vi "TSM Set AI Microphone DAQmx Tasks.vi"(0 "TSM context":T1, 5 "Sampling Rate (Hz)":dbl format="%#_6pHz", 7 "Samples per channel":i32=1000, 9 "max dB SPL":dbl=132.0 format="%.2p", 11 "error in (no error)":errorcluster) -> (15 "error out":errorcluster)   [LabVIEW 2020]
doc: "Use this VI to initialize AI tasks for Microphones on connected NI-DAQmx instruments in the pin map associated with the test program."
uses:
  <vilib>/NI_TestStand_SemiconductorModule/NI_TestStand_Semiconductor_Module.lvlibp/PinMap/General/SemiconductorModuleContext.ctl
  <vilib>/DAQmx/create/channels.llb/DAQmx Create Channel (AI-Sound Pressure-Microphone).vi
  <vilib>/DAQmx/configure/timing.llb/DAQmx Timing (Sample Clock).vi
  <vilib>/NI_TestStand_SemiconductorModule/NI_TestStand_Semiconductor_Module.lvlibp
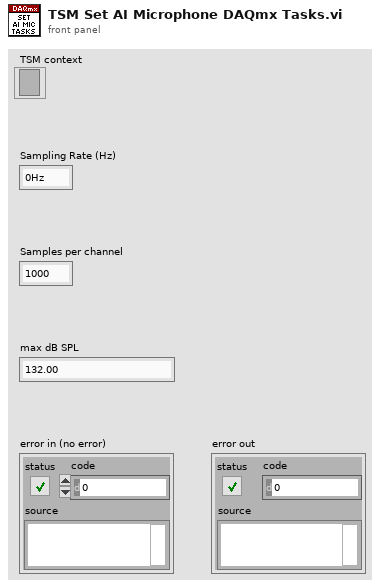
[diagram p1: front panel]
types:
  T1 = typedef "NI_TestStand_Semiconductor_Module.lvlibp/SemiconductorModuleContext.ctl" = refnum<k7>
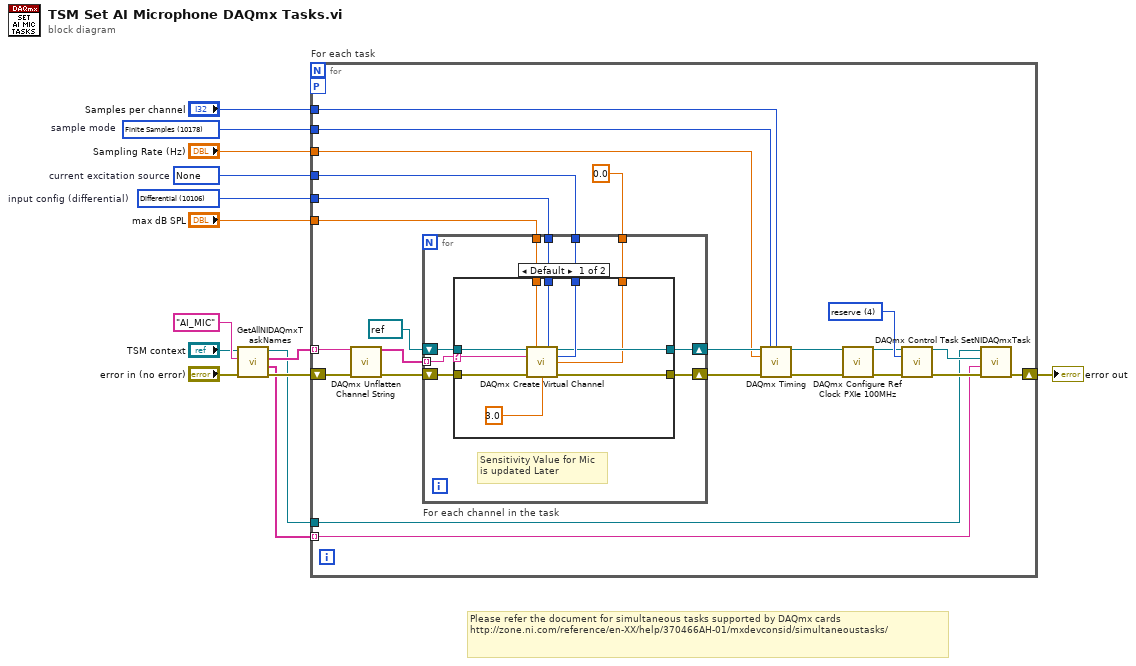
[diagram p0: block diagram]
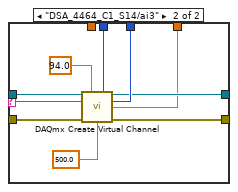
[diagram p2: hidden frame]
diagram:
  w1 = 10178 items=["Finite Samples"=10178, "Continuous Samples"=10123, "Hardware Timed Single Point"=12522]  # sample mode
  w10 = 10106 items=["default"=-1, "RSE"=10083, "NRSE"=10078, "Differential"=10106, "Pseudodifferential"=12529]  # input config (differential)
  w11 = 10230 items=["Internal"=10200, "External"=10167, "None"=10230]  # current excitation source
  # "Please refer the document for simultaneous tasks supported by DAQmx cards\nhttp://zone.ni.com/reference/en-XX/help/370466AH-01/mxdevconsid/simultaneoustasks/"
  n1 = call <vilib>:"GetAllNIDAQmxTaskNames.vi"("error in (no error)"="error in (no error)", "Task Type"="AI_MIC", "Semiconductor Module Context"="TSM context") -> ("error out"=w6:errorcluster, "Task Names"=w4:string[], "Channel Lists"=w7:string[], "Semiconductor Module Context Out"=w5:T1)  [unwired: 5 in]
  n2 = for "For each task" {
    tunnel: "max dB SPL" -> [w38]
    tunnel: w11 -> [w37]
    tunnel: w10 -> [w36]
    shift-right: [w25] -> w3
    shift-left: w6 -> [w35]
    tunnel: w7 -> [w19] mode=indexing
    tunnel: "Samples per channel" -> [w32]
    tunnel: "Sampling Rate (Hz)" -> [w31]
    tunnel: w5 -> [w27]
    tunnel: w4 -> [w26] mode=indexing
    workers-P: _ -> [_]
    tunnel: w1 -> [w16]
    w30 = 4 items=["verify"=2, "reserve"=4, "commit"=3, "unreserve"=5, "abort"=6] ("action")
    n3 = call <vilib>:"DAQmx Unflatten Channel String.vi"("names in"=w19, "error in"=w35) -> ("names out"=w18:string[], "error out"=w20:errorcluster)  [unwired: 12 in]
    n4 = for "For each channel in the task" {
      tunnel: w38 -> [w47]
      tunnel: w37 -> [w46]
      tunnel: w36 -> [w45]
      shift-right: [w44] -> w34
      shift-left: w20 -> [w42]
      tunnel: w18 -> [w40] mode=indexing
      shift-right: [w43] -> w33
      shift-left: refnum<k21> refnum ("task in") -> [w41]
      tunnel: 0.0 ("current excitation value") -> [w39]
      # "Sensitivity Value for Mic\nis updated Later"
      n5 = case shown="Default" w40 {
        selector: w40 -> [w50 w61]
        tunnel: w47 -> [w57 _]
        tunnel: w46 -> [w56 w67]
        tunnel: w45 -> [w55 w66]
        tunnel: [w54 w65] -> w44
        tunnel: [w53 w64] -> w43
        tunnel: w42 -> [w52 w63]
        tunnel: w41 -> [w51 w62]
        tunnel: w39 -> [w49 w60]
        frame Default {
          n6 = call-poly <vilib>:"DAQmx Create Virtual Channel.vi"("task in"=w51, "maximum sound pressure level"=w57, "input terminal configuration"=w55, "physical channels"=w50, "current excitation source"=w56, "current excitation value"=w49, "error in"=w52, "microphone sensitivity"=3.0) -> ("task out"=w53:refnum<k21>, "error out"=w54:errorcluster)  [unwired: 6 in]
        }
        frame "DSA_4464_C1_S14/ai3" {
          n7 = call-poly <vilib>:"DAQmx Create Virtual Channel.vi"("task in"=w62, "maximum sound pressure level"=94.0, "input terminal configuration"=w66, "physical channels"=w61, "current excitation source"=w67, "current excitation value"=w60, "error in"=w63, "microphone sensitivity"=500.0) -> ("task out"=w64:refnum<k21>, "error out"=w65:errorcluster)  [unwired: 6 in]
        }
      }
    }
    n8 = call-poly <vilib>:"DAQmx Timing.vi"("task/channels in"=w33, "sample mode"=w16, "samples per channel"=w32, "rate"=w31, "error in"=w34) -> ("task out"=w24:refnum<k21>, "error out"=w23:errorcluster)  [unwired: 9 in]
    n9 = call "DAQmx Configure Ref Clock PXIe 100MHz.vi"("DAQmx Task In"=w24, "error in (no error)"=w23) -> ("DAQmx Task Out"=w22:refnum<k21>, "error out"=w21:errorcluster)  [unwired: 12 in]
    n10 = call <vilib>:"DAQmx Control Task.vi"("task/channels in"=w22, "action"=w30, "error in"=w21) -> ("task out"=w28:refnum<k21>, "error out"=w29:errorcluster)  [unwired: 11 in]
    n11 = call <vilib>:"SetNIDAQmxTask.vi"("error in (no error)"=w29, "Task Name"=w26, "DAQmx Task"=w28, "Semiconductor Module Context"=w27) -> ("error out"=w25:errorcluster)  [unwired: 6 in, 1 out]
  }
  "error out" <- w3
